vi "List_Files.vi"(8 "error in (no error)":errorcluster, 11 "IB_Source in":refnum<class "IB_Source.lvclass">) -> (0 "error out":errorcluster, 3 "Files":T1[](array[typedef]))   [LabVIEW 2020, in "IB_Source.lvclass"]
uses:
  <vilib>/AppBuilder/IB_Classes/Source/IB_Source.lvclass
  <vilib>/AppBuilder/IB_Classes/Source/IB_Source.lvclass/IB_Source.ctl
  <vilib>/AppBuilder/IB_Classes/Source/File/IB_Source_File.lvclass
  <resource>/Framework/Providers/Builds/Installer/CDK_sTypeDef_FileList.ctl
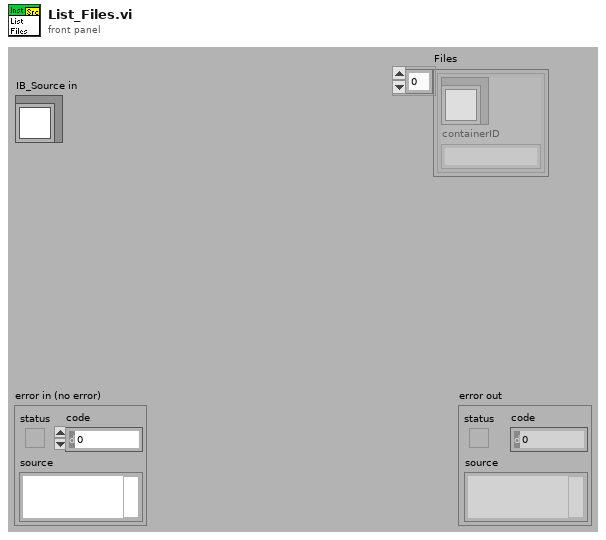
[diagram p1: front panel]
types:
  T1 = typedef "CDK_sTypeDef_FileList.ctl" = cluster{"FileInventory":refnum<class "IB_Source_File.lvclass">, "containerID":string}
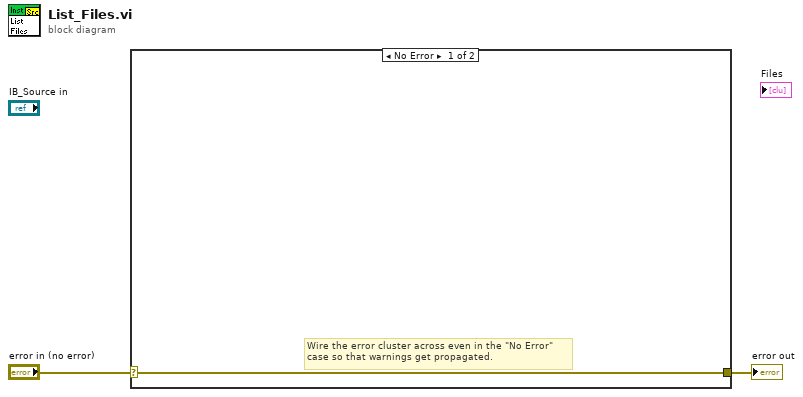
[diagram p0: block diagram]
diagram:
  n1 = case shown="No Error" "error in (no error)" {
    selector: "error in (no error)" -> [w3 w4]
    tunnel: [w3 w4] -> w1
    frame No Error {
      # "Wire the error cluster across even in the \"No Error\"\ncase so that warnings get propagated."
    }
    frame Error {
    }
  }
  "error out" <- w1
